vi "Yokogawa WT1800 Series Measure Harmonics Preset.vi"() -> ()   [LabVIEW 2015]
doc: "This example shows how to measure the harmonic measurement numeric preset list data\n\n<b>Note:</b>\nThis setting valid on models with the harmonic measurement (/G5 or /G6) option."
uses:
  <instrlib>/Yokogawa WT1800 Series/Public/Data/Low Level/Fetch Measurement (Harmonics).vi
  <instrlib>/Yokogawa WT1800 Series/Yokogawa WT1800 Series.lvlib
panel:
  in  "Preset (Pattern 1)":i32(ring)=1 items=["Pattern 1"=1, "Pattern 2"=2, "Pattern 3"=3, "Pattern 4"=4]
  out "Measurement":dbl[][](array[numeric])
  out "Function":string[](array[string])
  in  "Number of Item (15)":i32=15 min=1 max=64
  in  "Timeout (10000 ms)":i32=10000 min=1
  in  "VISA resource name":refnum<visa-resource-name>
  # "(c) 2011 Yokogawa Meters & Instruments Corporation.  All rights reserved."
  # "WT1800 SERIES POWER ANALYZER"
  # "Total        DC            1             2              3             4"
  # "ms"
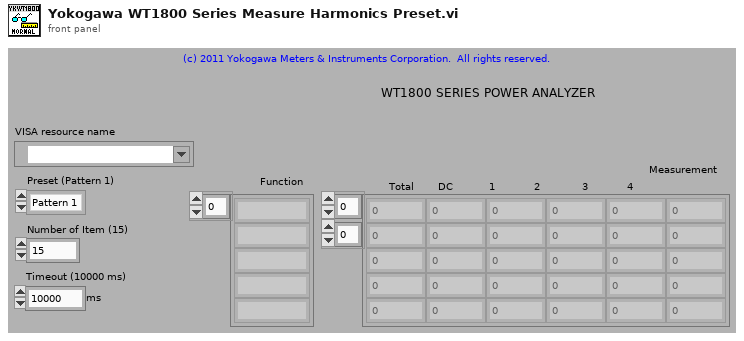
[diagram p1: front panel]
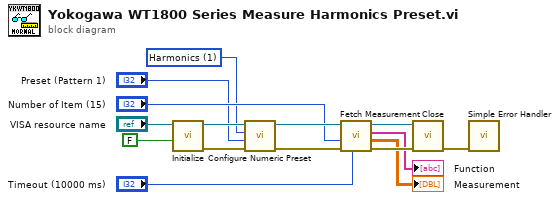
[diagram p0: block diagram]
diagram:
  w1 = 1 items=["Normal", "Harmonics"] ("Target Item (0: Normal)")
  n1 = call <instrlib>:"Initialize.vi"("Reset (True)"=FALSE ("Reset? (True)"), "VISA resource name"="VISA resource name") -> ("error out"=w4:errorcluster, "VISA resource name out"=w5:refnum<visa-resource-name>)  [unwired: 8 in]
  n2 = call <instrlib>:"Configure Numeric Preset.vi"("error in (no error)"=w4, "Preset (Pattern 1)"="Preset (Pattern 1)", "Target Item (0: Normal)"=w1, "VISA resource name"=w5) -> ("error out"=w9:errorcluster, "VISA resource name out"=w10:refnum<visa-resource-name>)  [unwired: 6 in]
  n3 = call-poly <instrlib>:"Fetch Measurement.vi"("Timeout (10000 ms)"="Timeout (10000 ms)", "error in (no error)"=w9, "Number of Item (15)"="Number of Item (15)", "VISA resource name"=w10) -> ("error out"=w12:errorcluster, "Measurement"=→"Measurement":dbl[][], "Function"=→"Function":string[], "VISA resource name out"=w13:refnum<visa-resource-name>)  [unwired: 4 in]
  n4 = call <instrlib>:"Close.vi"("error in (no error)"=w12, "VISA resource name"=w13) -> ("error out"=w15:errorcluster)  [unwired: 9 in]
  n5 = call <vilib>:"Simple Error Handler.vi"("error in (no error)"=w15) -> ()  [unwired: 4 in, 5 out]
